vi "Radians to Degrees (Scalar EXT).vi"(3 "angle (rad)":ext caption="角（弧度）") -> (1 "angle (deg)":ext caption="角（角度）")   [LabVIEW 2011, in "NI_AngleManipulation.lvlib"]
doc: "Converts an angle from radians to degrees."
uses:
  <vilib>/Utility/AngleManip/NI_AngleManipulation.lvlib
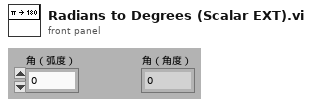
[diagram p1: front panel]
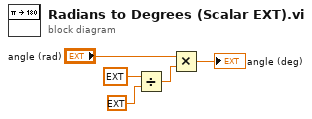
[diagram p0: block diagram]
diagram:
  n1 = Divide(x=ext 180.0 ("y"), y=ext 3.1415926535897932385) -> (x/y=w2:ext)
  n2 = Multiply(x="angle (rad)", y=w2) -> (x*y=→"angle (deg)":ext)
